vi "Start Log.vi"(8 "error in (no error)":errorcluster, 10 "Test Series":string, 11 "DemoApp in":refnum<class "DemoApp.lvclass">) -> (0 "error out":errorcluster, 3 "DemoApp out":refnum<class "DemoApp.lvclass">)   [LabVIEW 2020, in "VolatusDemo.lvlib" / "DemoApp.lvclass"]
uses:
  DemoApp.lvclass
  Volatus/LoggingAPI/LoggingAPI.lvclass
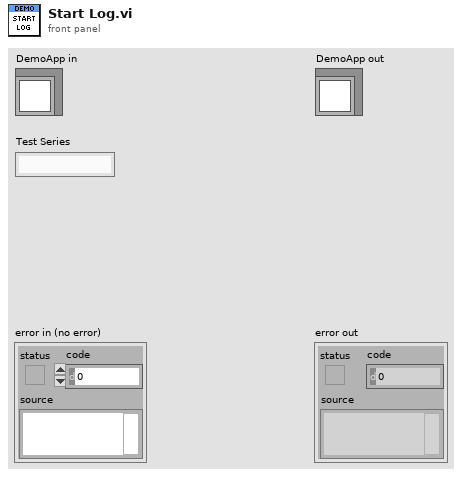
[diagram p1: front panel]
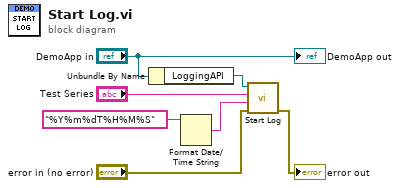
[diagram p0: block diagram]
diagram:
  n1 = Unbundle By Name("DemoApp in") -> ("LoggingAPI"=w6:refnum<class "LoggingAPI.lvclass">)
  n2 = Format Date/Time String(time format string (%c)="%Y%m%dT%H%M%S" ("format string")) -> (date/time string=w1:string)  [unwired: 2 in]
  n3 = call "Start Log.vi"("error in (no error)"="error in (no error)", "Timestamp"=w1, "Series"="Test Series", "LoggingAPI in"=w6) -> ("error out"=→"error out":errorcluster)  [unwired: 6 in, 1 out]
  "DemoApp out" <- "DemoApp in"
